vi "Get Component Settings By ID.vi"(8 "error in (no error)":errorcluster, 10 "settings id":T1={"plugin"=-1, "thread"=-1, "group"=-1, "transfer"=-1, "channel"=-1}, 11 "Group Configuration in":refnum<class "Group Configuration.lvclass">) -> (0 "error out":errorcluster, 2 "component settings":T2[](array[typedef]), 3 "Group Configuration out":refnum<class "Group Configuration.lvclass">)   [LabVIEW 2019, in "DSF Core.lvlib" / "Group Configuration.lvclass"]
uses:
  Group Configuration.lvclass
  C:/Dev/GitHub/niveristand-data-sharing-framework-custom-device/Core/Classes/Configuration/Core/Core Configuration.lvclass
  Typedefs/DSF Settings Info.ctl
  Typedefs/DSF Configuration ID.ctl
  Group Configuration.lvclass/Group Configuration.ctl
  Transfer/Transfer Configuration.lvclass
  Core Configuration.lvclass
  DSF Core.lvlib
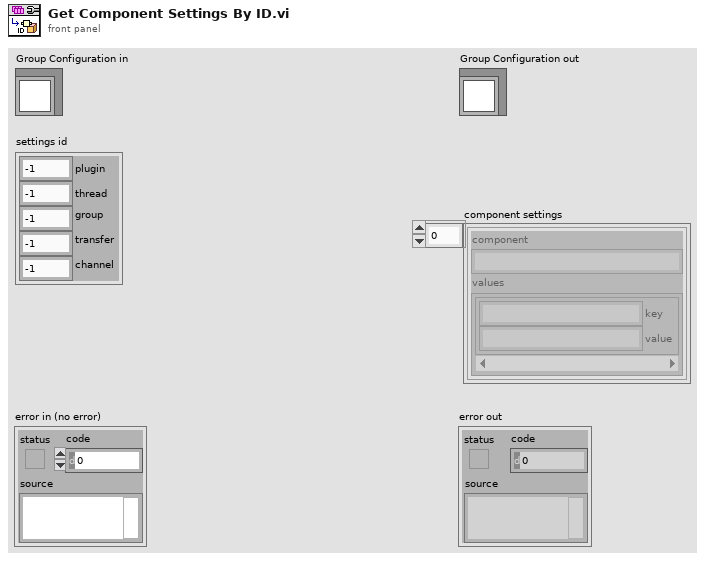
[diagram p1: front panel]
types:
  T1 = typedef "DSF Core.lvlib/DSF Configuration ID.ctl" = cluster{"plugin":i32, "thread":i32, "group":i32, "transfer":i32, "channel":i32}
  T2 = typedef "DSF Core.lvlib/DSF Settings Info.ctl" = cluster{"component":string, "values":cluster{"key":string, "value":string}[]}
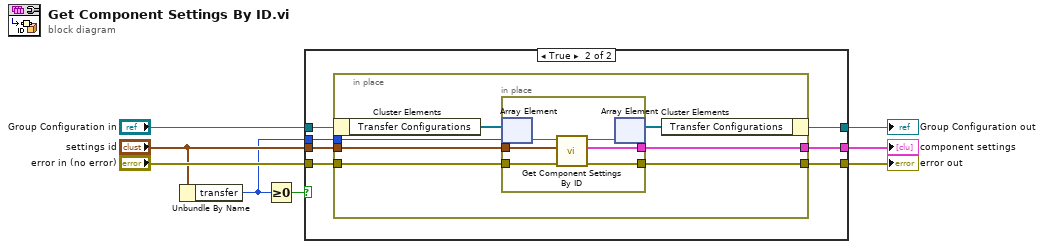
[diagram p0: block diagram]
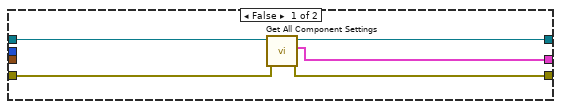
[diagram p2: hidden frame]
diagram:
  n1 = Unbundle By Name("settings id") -> ("transfer"=w1:i32)
  n2 = Greater Or Equal To 0?(x=w1) -> (x >= 0?=w8:bool)
  n3 = case shown="True" w8 {
    tunnel: [w11 w14] -> w2
    tunnel: w1 -> [_ w16]
    tunnel: "error in (no error)" -> [w12 w20]
    tunnel: [w10 w19] -> w6
    tunnel: [w9 w18] -> w5
    tunnel: "settings id" -> [_ w17]
    tunnel: "Group Configuration in" -> [w13 w15]
    frame False {
      n4 = call "Get All Component Settings.vi"("error in (no error)"=w12, "Runtime Configuration in"=w13) -> ("error out"=w10:errorcluster, "component settings"=w9:T2[], "Runtime Configuration out"=w11:refnum<class "Group Configuration.lvclass">)  [unwired: 7 in]
    }
    frame True {
      n5 = in-place {
        in-place-border: w20 -> [w27]
        in-place-border: [w26] -> w19
        in-place-border: [w25] -> w18
        in-place-border: w17 -> [w24]
        in-place-border: w16 -> [w23]
        n6 = in-place-cluster #1(w15) -> ("Transfer Configurations"=w22:refnum<class "Transfer Configuration.lvclass">[])
        n7 = in-place {
          in-place-border: w27 -> [w33]
          in-place-border: [w32] -> w26
          in-place-border: [w31] -> w25
          in-place-border: w24 -> [w30]
          n8 = in-place-array #2(w22, w23) -> (w29:refnum<class "Transfer Configuration.lvclass">)
          n9 = call-dynamic "Get Component Settings By ID.vi"("error in (no error)"=w33, "settings id"=w30, "Transfer Configuration in"=w29) -> ("error out"=w32:errorcluster, "component settings"=w31:T2[], "Transfer Configuration out"=w28:refnum<class "Transfer Configuration.lvclass">)  [unwired: 6 in]
          n10 = in-place-array #2(w28) -> (w21:refnum<class "Transfer Configuration.lvclass">[])  [unwired: 1 out]
        }
        n11 = in-place-cluster #1("Transfer Configurations"=w21) -> (w14:refnum<class "Group Configuration.lvclass">)
      }
    }
  }
  "error out" <- w6
  "Group Configuration out" <- w2
  "component settings" <- w5
